vi "Unflatten Value.vi"(8 "Error In":errorcluster, 10 "Value":string, 11 "Path In":refnum<class "Path.lvclass">) -> (0 "Error Out":errorcluster, 3 "Path Out":refnum<class "Path.lvclass">)   [LabVIEW 2020, in "NI_VIAnCFGDataStructure.lvlib" / "Path.lvclass"]
uses:
  <vilib>/addons/analyzer/VIAnCFGDataStructure/Data Types/Path/Path.lvclass
  <vilib>/addons/analyzer/VIAnCFGDataStructure/Data Types/Path/Path.lvclass/Path.ctl
  <vilib>/addons/analyzer/VIAnCFGDataStructure/Tree Manager/API/Generate Hash.vi
  <vilib>/addons/analyzer/VIAnCFGDataStructure/Tree Manager/Tree.lvclass
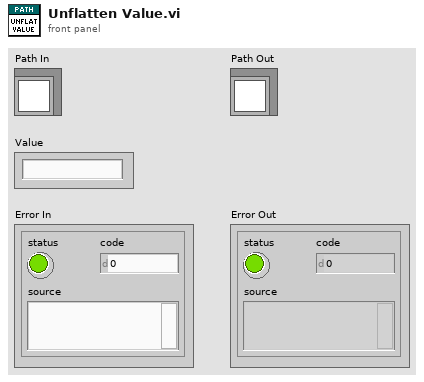
[diagram p1: front panel]
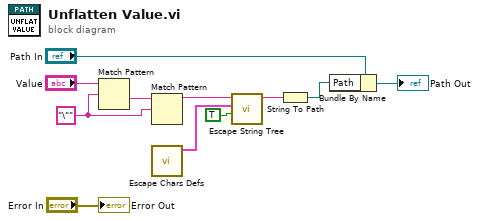
[diagram p0: block diagram]
diagram:
  w5 = "\"" ("regular expression")
  n1 = Match Pattern(string="Value", regular expression=w5) -> (after substring=w6:string)  [unwired: 1 in, 3 out]
  n2 = Match Pattern(string=w6, regular expression=w5) -> (before substring=w3:string)  [unwired: 1 in, 3 out]
  n3 = call <vilib>:"Escape Chars Defs.vi"() -> ("Escapes"=w4:cluster{"String":string, "Escape":string}[])  [unwired: 11 in]
  n4 = call <vilib>:"Escape String Tree.vi"("Reverse? (False)"=TRUE, "Escapes"=w4, "String In"=w3) -> ("String Out"=w1:string)  [unwired: 8 in]
  n5 = String To Path(string=w1) -> (path=w9:path)
  n6 = Bundle By Name(cluster="Path In", "Path"=w9) -> (→"Path Out":refnum<class "Path.lvclass">)
  "Error Out" <- "Error In"
